vi "Read HW Parameters.vi"(7 "Pump ID (0:A)":T2, 8 "error in (no error)":errorcluster, 11 "VISA Refnum in":refnum<visa-resource-name>) -> (0 "error out":errorcluster, 2 "Hardware Configuration":T1={"Head type"=enum."High Flow", "Pressure range"=enum."High pressure", "Stator material"=enum."PTFE", "Rotor material"=enum."Ceramic", "Rotor O-ring material"=enum."none", "Piston O-ring material"=enum."Viton", "Pump body material"=enum."Stainless steel", "Controller"=enum."MForce", "Gear ratio"=enum."9.87", "Motor resolution"=enum."1.8", "Equipped with encoder"=enum."No"}, 3 "VISA Refnum out":refnum<visa-resource-name>)   [LabVIEW 2020, in "Global FIA milliGAT.lvlib"]
uses:
  <instrlib>/RxnRover/Global FIA milliGAT 3.14/Global FIA milliGAT.lvlib
  <instrlib>/RxnRover/Global FIA milliGAT 3.14/Public/Utility/Pump Address.ctl
  <instrlib>/RxnRover/Global FIA milliGAT 3.14/Public/Utility/Low Level/Hardware Configuration.ctl
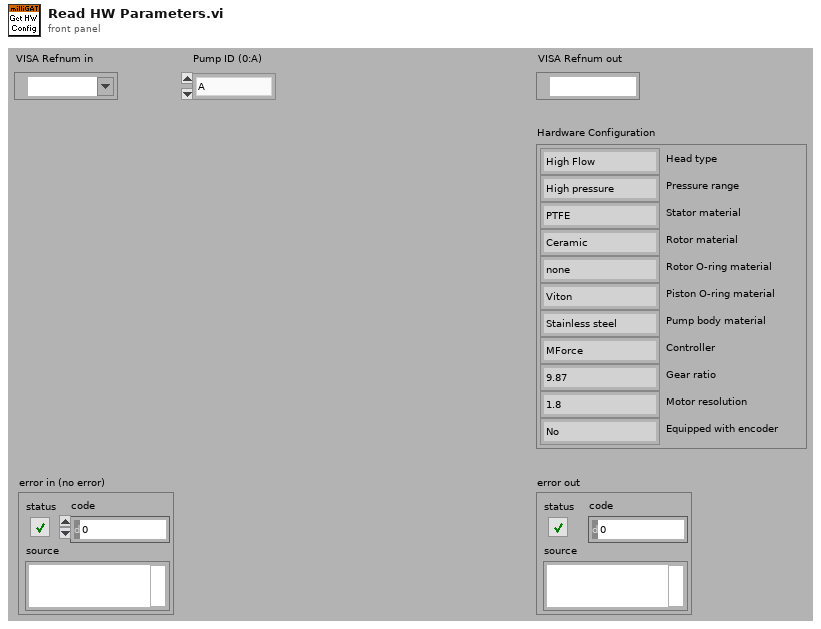
[diagram p1: front panel]
types:
  T1 = typedef "Global FIA milliGAT.lvlib/Hardware Configuration.ctl" = cluster{"Head type":enum16{"Low Flow", "High Flow"}, "Pressure range":enum16{"Low pressure", "High pressure"}, "Stator material":enum16{"PTFE", "Valcon E3", "PEEK/PTFE", "Valcon H2"}, "Rotor material":enum16{"Ceramic", "Valcon P", "CTFE"}, "Rotor O-ring material":enum16{"none", "Viton", "Kalrez"}, "Piston O-ring material":enum16{"Viton", "Kalrez"}, "Pump body material":enum16{"Stainless steel", "Aluminum"}, "Controller":enum16{"MForce", "MDrive"}, "Gear ratio":enum16{"4.75", "9.87", "15", "22.56"}, "Motor resolution":enum16{"1.8", "0.9"}, "Equipped with encoder":enum16{"No", "Yes"}}
  T2 = typedef "Global FIA milliGAT.lvlib/Pump Address.ctl" = enum16{"A", "B", "C", "D", "E", "F", "G", "H", "I", "J", "K", "L", "M", "N", "O", "P", "Q", "R", "S", "T", "U", "V", "W", "X", "Y", "Z", "a", "b", "c", "d", "e", "f", "g", "h", "i", "j", "k", "l", "m", "n", "o", "p", "q", "r", "s", "t", "u", "v", "w", "x", "y", "z", "0", "1", "2", "3", "4", "5", "6", "7", "8", "9"}
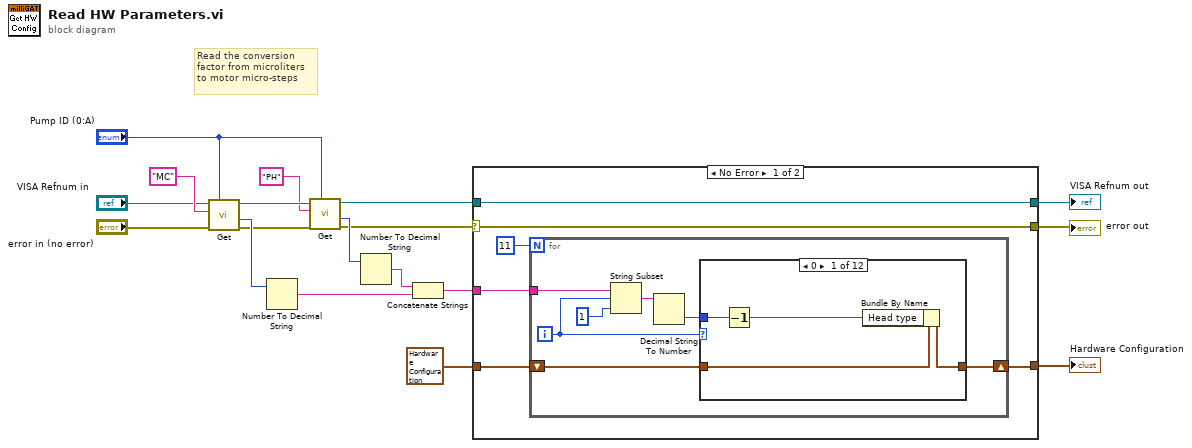
[diagram p0: block diagram]
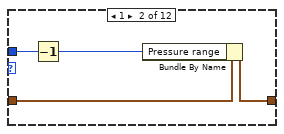
[diagram p2: hidden frame]
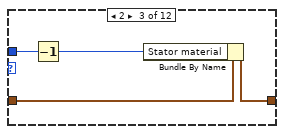
[diagram p3: hidden frame]
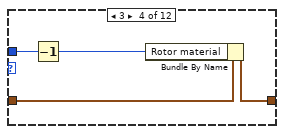
[diagram p4: hidden frame]
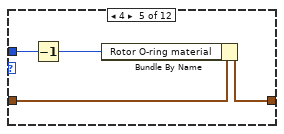
[diagram p5: hidden frame]
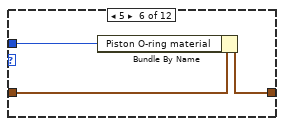
[diagram p6: hidden frame]
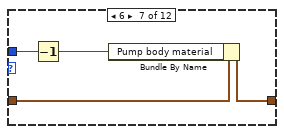
[diagram p7: hidden frame]
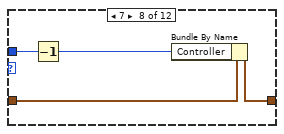
[diagram p8: hidden frame]
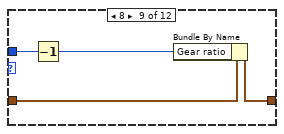
[diagram p9: hidden frame]
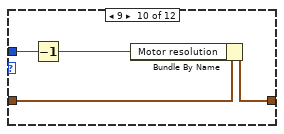
[diagram p10: hidden frame]
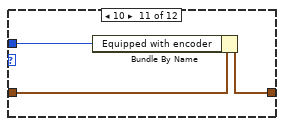
[diagram p11: hidden frame]
diagram:
  # "Read the conversion\nfactor from microliters\nto motor micro-steps"
  n1 = call <instrlib>:"Get.vi"("Pump ID (0:A)"="Pump ID (0:A)", "error in (no error)"="error in (no error)", "Parameter"="MC" ("Parameter Name"), "VISA resource in"="VISA Refnum in") -> ("error out"=w13:errorcluster, "Value"=w15:i32, "VISA resource out"=w12:refnum<visa-resource-name>)  [unwired: 5 in]
  n2 = Number To Decimal String(number=w15) -> (decimal integer string=w17:string)  [unwired: 1 in]
  n3 = call <instrlib>:"Get.vi"("Pump ID (0:A)"="Pump ID (0:A)", "error in (no error)"=w13, "Parameter"="PH" ("Parameter Name"), "VISA resource in"=w12) -> ("error out"=w9:errorcluster, "Value"=w14:i32, "VISA resource out"=w8:refnum<visa-resource-name>)  [unwired: 5 in]
  n4 = Number To Decimal String(number=w14) -> (decimal integer string=w16:string)  [unwired: 1 in]
  n5 = Concatenate Strings(w16, w17) -> (w18:string)
  n6 = case shown="No Error" w9 {
    selector: w9 -> [w20 w76]
    tunnel: w18 -> [w24 _]
    tunnel: w8 -> [w19 w77]
    tunnel: [w19 w77] -> w6
    tunnel: [w20 w76] -> w7
    tunnel: T1 {"Head type"=enum."Low Flow", "Pressure range"=enum."Low pressure", "Stator material"=enum."PTFE", "Rotor material"=enum."Ceramic", "Rotor O-ring material"=enum."none", "Piston O-ring material"=enum."Viton", "Pump body material"=enum."Stainless steel", "Controller"=enum."MForce", "Gear ratio"=enum."4.75", "Motor resolution"=enum."1.8", "Equipped with encoder"=enum."No"} ("Hardware Configuration") -> [w22 w75]
    tunnel: [w21 w75] -> w1
    frame No Error {
      n7 = for {
        N: 11 -> [_]
        tunnel: w24 -> [w31]
        shift-right: [w25] -> w21
        shift-left: w22 -> [w26]
        i -> [w30]
        n8 = String Subset(string=w31, offset (0)=w30, length (rest)=1 ("length (rest)")) -> (substring=w29:string)
        n9 = Decimal String To Number(string=w29) -> (number=w28:i32)  [unwired: 2 in, 1 out]
        n10 = case shown="0" w30 {
          tunnel: w28 -> [w35 w39 w43 w47 w51 w52 w58 w62 w66 w70 w71 _]
          tunnel: w26 -> [w34 w37 w41 w45 w49 w53 w56 w60 w64 w68 w72 w74]
          tunnel: [w33 w38 w42 w46 w50 w54 w57 w61 w65 w69 w73 w74] -> w25
          frame 0 {
            n11 = Decrement(x=w35) -> (x-1=w32:i32)
            n12 = Bundle By Name(cluster=w34, "Head type"=w32) -> (w33:T1)
          }
          frame 1 {
            n13 = Decrement(x=w39) -> (x-1=w36:i32)
            n14 = Bundle By Name(cluster=w37, "Pressure range"=w36) -> (w38:T1)
          }
          frame 2 {
            n15 = Decrement(x=w43) -> (x-1=w40:i32)
            n16 = Bundle By Name(cluster=w41, "Stator material"=w40) -> (w42:T1)
          }
          frame 3 {
            n17 = Decrement(x=w47) -> (x-1=w44:i32)
            n18 = Bundle By Name(cluster=w45, "Rotor material"=w44) -> (w46:T1)
          }
          frame 4 {
            n19 = Decrement(x=w51) -> (x-1=w48:i32)
            n20 = Bundle By Name(cluster=w49, "Rotor O-ring material"=w48) -> (w50:T1)
          }
          frame 5 {
            n21 = Bundle By Name(cluster=w53, "Piston O-ring material"=w52) -> (w54:T1)
          }
          frame 6 {
            n22 = Decrement(x=w58) -> (x-1=w55:i32)
            n23 = Bundle By Name(cluster=w56, "Pump body material"=w55) -> (w57:T1)
          }
          frame 7 {
            n24 = Decrement(x=w62) -> (x-1=w59:i32)
            n25 = Bundle By Name(cluster=w60, "Controller"=w59) -> (w61:T1)
          }
          frame 8 {
            n26 = Decrement(x=w66) -> (x-1=w63:i32)
            n27 = Bundle By Name(cluster=w64, "Gear ratio"=w63) -> (w65:T1)
          }
          frame 9 {
            n28 = Decrement(x=w70) -> (x-1=w67:i32)
            n29 = Bundle By Name(cluster=w68, "Motor resolution"=w67) -> (w69:T1)
          }
          frame 10 {
            n30 = Bundle By Name(cluster=w72, "Equipped with encoder"=w71) -> (w73:T1)
          }
          frame Default {
          }
        }
      }
    }
    frame Error {
    }
  }
  "VISA Refnum out" <- w6
  "error out" <- w7
  "Hardware Configuration" <- w1
